vi "Read.vi"(8 "error in (no error)":errorcluster, 10 "Timeout(10000 ms)":u32=10000, 11 "VISA resource name":refnum<visa-resource-name>) -> (0 "error out":errorcluster, 1 "Measurements Metadata":T1(array[cluster]), 2 "Measurements":dbl[](array[numeric]), 3 "VISA resource name out":refnum<visa-resource-name>)   [LabVIEW 2021, in "Keithley 2182.lvlib"]
doc: "Performs the following:\n\n1. <B>Abort:</B> The instrument goes into the idle state if continuous initiation is disabled. If continuous initiation is enabled, the operation re-starts at the beginning of the Trigger Model.\n2. <B>Inititate:</B> If the instrument is in the idle state, Initiate takes the instrument out of the idle state. If continuous initiation is enabled (Continuous is selected in Intiate VI) then the Initiate generates an error and ignores the command.\n3. <B>Fetch:</B> Reads the measurements generated from the Initate.\n\nThis VI is typically used with the instrument in the \"one-shot\" measurement mode to\ntrigger and acquire a specified number of readings. The <B>Configure Measurements</B> VI is used to specify the number of readings.\n\n<B>Note:</B>\n1. The readings are stored in the buffer.\n2. You cannot use this VI if sample count > 1 and there are readings stored in the buffer. Either set sample count to 1 or clear the buffer."
uses:
  <instrlib>/Keithley 2182/Keithley 2182.lvlib
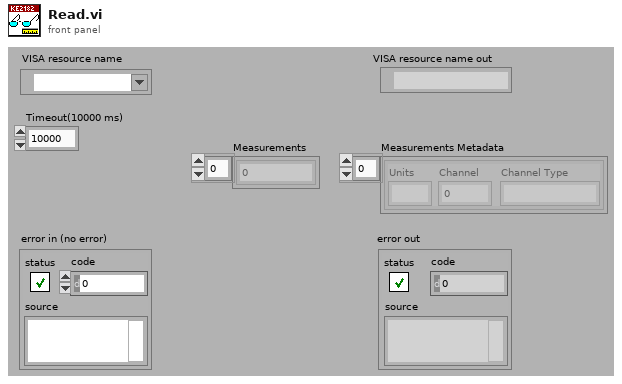
[diagram p1: front panel]
types:
  T1 = cluster{"Units":string, "Channel":i32, "Channel Type":string}[]
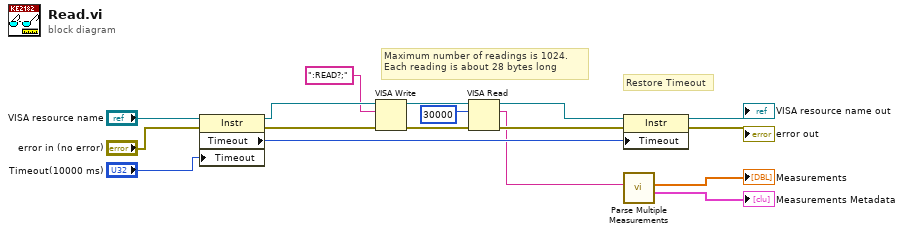
[diagram p0: block diagram]
diagram:
  # "Maximum number of readings is 1024.\nEach reading is about 28 bytes long"
  # "Restore Timeout"
  n1 = property class="Instr"(reference="VISA resource name", error in="error in (no error)", "Timeout"="Timeout(10000 ms)") -> (reference out=w14:refnum<visa-resource-name>, error out=w15:errorcluster, "Timeout"=w6:u32)
  n2 = VISA Write(VISA resource name=w14, write buffer=":READ?;", error in (no error)=w15) -> (VISA resource name out=w12:refnum<visa-resource-name>, error out=w11:errorcluster)  [unwired: 1 out]
  n3 = VISA Read(VISA resource name=w12, byte count=u32 30000, error in (no error)=w11) -> (VISA resource name out=w5:refnum<visa-resource-name>, read buffer=w3:string, error out=w4:errorcluster)  [unwired: 1 out]
  n4 = property class="Instr"(reference=w5, error in=w4, "Timeout"=w6) -> (reference out=→"VISA resource name out":refnum<visa-resource-name>, error out=→"error out":errorcluster)
  n5 = call <instrlib>:"Parse Multiple Measurements.vi"("Measurement String"=w3) -> ("Measurements Metadata"=→"Measurements Metadata":T1, "Measurements"=→"Measurements":dbl[])  [unwired: 9 in]
